vi "Calculate Frames per Second.vi"(9 "Reset":bool, 10 "Update Interval (ms)":u32=1000, 11 "Buffer Number":u32) -> (1 "Missed Frames":bool, 2 "Processed Frames/s":dbl, 3 "Acquired Frames/s":dbl)   [LabVIEW 2012]
doc: "Calculate the frame rate from within a loop. Frame rate is averaged over the specified update interval. The default update interval is 1000ms."
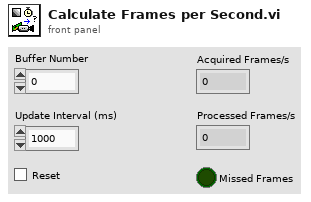
[diagram p1: front panel]
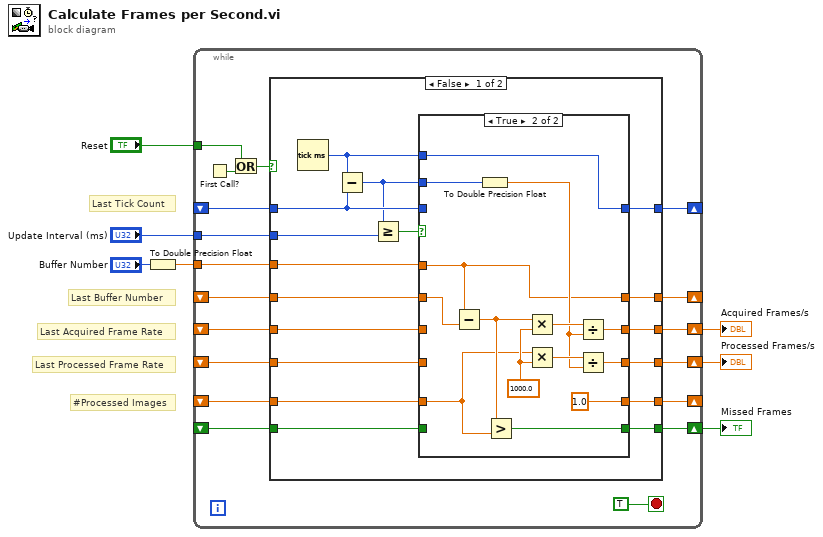
[diagram p0: block diagram]
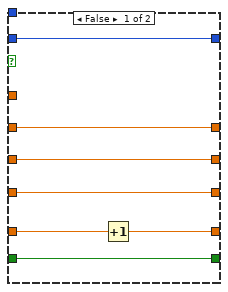
[diagram p2: hidden frame]
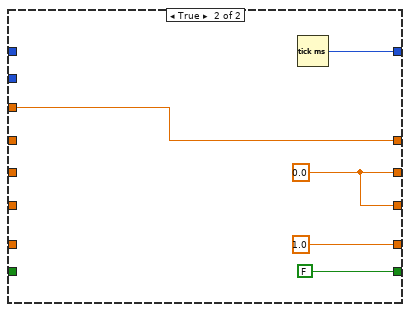
[diagram p3: hidden frame]
diagram:
  # "Last Processed Frame Rate"
  # "#Processed Images"
  # "Last Buffer Number"
  # "Last Acquired Frame Rate"
  # "Last Tick Count"
  n1 = To Double Precision Float(number="Buffer Number") -> (double precision float=w2:dbl)
  n2 = while {
    shift-right: [w24] -> _
    shift-left: _ -> [w23]
    shift-right: [w21] -> _
    shift-left: _ -> [w22]
    shift-right: [w20] -> w7
    shift-left: _ -> [w19]
    shift-right: [w18] -> _
    shift-left: _ -> [w17]
    shift-right: [w16] -> w6
    shift-left: _ -> [w15]
    tunnel: "Update Interval (ms)" -> [w14]
    tunnel: w2 -> [w10]
    tunnel: "Reset" -> [w9]
    shift-right: [w13] -> w4
    shift-left: _ -> [w8]
    stop <- TRUE stop-if-true
    n3 = First Call?() -> (First Call?: T/F=w12:bool)
    n4 = Or(x=w9, y=w12) -> (x .or. y?=w11:bool)
    n5 = case shown="False" w11 {
      tunnel: [w40 w68] -> w24
      tunnel: w23 -> [w41 _]
      tunnel: w22 -> [w39 _]
      tunnel: [w38 w67] -> w21
      tunnel: [w35 w65] -> w20
      tunnel: w19 -> [w34 _]
      tunnel: w10 -> [w33 w67]
      tunnel: [w31 1.0 ("buffer number")] -> w18
      tunnel: w17 -> [w32 _]
      tunnel: [w30 w65] -> w16
      tunnel: w15 -> [w29 _]
      tunnel: w14 -> [w28 _]
      tunnel: [w27 FALSE] -> w13
      tunnel: w8 -> [w26 _]
      frame False {
        n6 = Tick Count (ms)() -> (millisecond timer value=w37:u32)
        n7 = Subtract(x=w37, y=w41) -> (x-y=w36:u32)
        n8 = Greater Or Equal?(x=w36, y=w28) -> (x >= y?=w42:bool)
        n9 = case shown="True" w42 {
          tunnel: w41 -> [w49 _]
          tunnel: [w49 w63] -> w40
          tunnel: w39 -> [w47 w60]
          tunnel: [w47 w51] -> w38
          tunnel: w37 -> [_ w63]
          tunnel: w36 -> [_ w56]
          tunnel: [w48 w61] -> w35
          tunnel: w34 -> [w48 _]
          tunnel: w33 -> [_ w51]
          tunnel: w32 -> [w46 w50]
          tunnel: [w45 1.0] -> w31
          tunnel: [w44 w55] -> w30
          tunnel: w29 -> [w44 _]
          tunnel: [w43 w52] -> w27
          tunnel: w26 -> [w43 _]
          frame False {
            n10 = Increment(x=w46) -> (x+1=w45:dbl)
          }
          frame True {
            w58 = 1000.0 ("y")
            n11 = Subtract(x=w51, y=w60) -> (x-y=w53:dbl)
            n12 = To Double Precision Float(number=w56) -> (double precision float=w54:dbl)
            n13 = Greater?(x=w53, y=w50) -> (0:w52:bool)
            n14 = Multiply(x=w53, y=w58) -> (x*y=w62:dbl)
            n15 = Multiply(x=w50, y=w58) -> (x*y=w57:dbl)
            n16 = Divide(x=w62, y=w54) -> (x/y=w61:dbl)
            n17 = Divide(x=w57, y=w54) -> (x/y=w55:dbl)
          }
        }
      }
      frame True {
        w65 = 0.0
        n18 = Tick Count (ms)() -> (millisecond timer value=w68:u32)
      }
    }
  }
  "Acquired Frames/s" <- w7
  "Processed Frames/s" <- w6
  "Missed Frames" <- w4
